vi "Connect.vi"(8 "error in (no error)":errorcluster, 11 "PicoScope 3000a in":refnum<class "PicoScope 3000a.lvclass">) -> (0 "error out":errorcluster, 3 "PicoScope 3000a out":refnum<class "PicoScope 3000a.lvclass">)   [LabVIEW 2018, in "PicoScope 3000a.lvlib" / "PicoScope 3000a.lvclass"]
doc: "This Override method is used initiative the communication session with the Oscope instrument."
uses:
  PicoScope 3000a.lvclass
  PicoScope 3000a.lvclass/PicoScope 3000a.ctl
  ps3000a.dll
  LWS SLA-070/Distro/Projects/12170 Luminar LWS Base/Source/PPLs/Oscilloscope.lvlibp/Oscilloscope.lvclass
  C:/Projects/LWS SLA-070/Distro/Projects/12170 Luminar LWS Base/Source/PPLs/Oscilloscope.lvlibp/Oscilloscope.lvclass
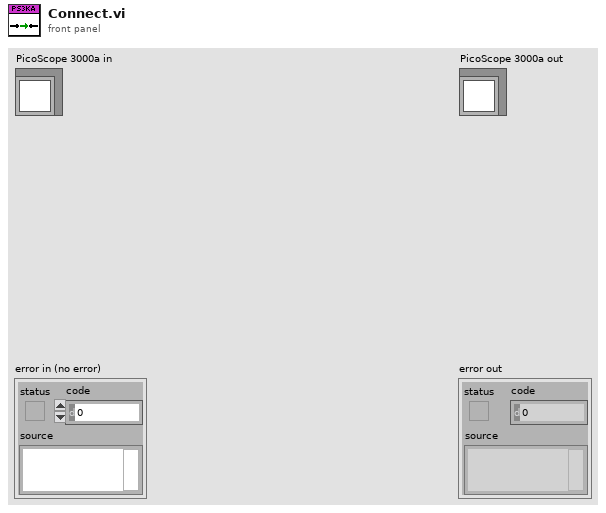
[diagram p1: front panel]
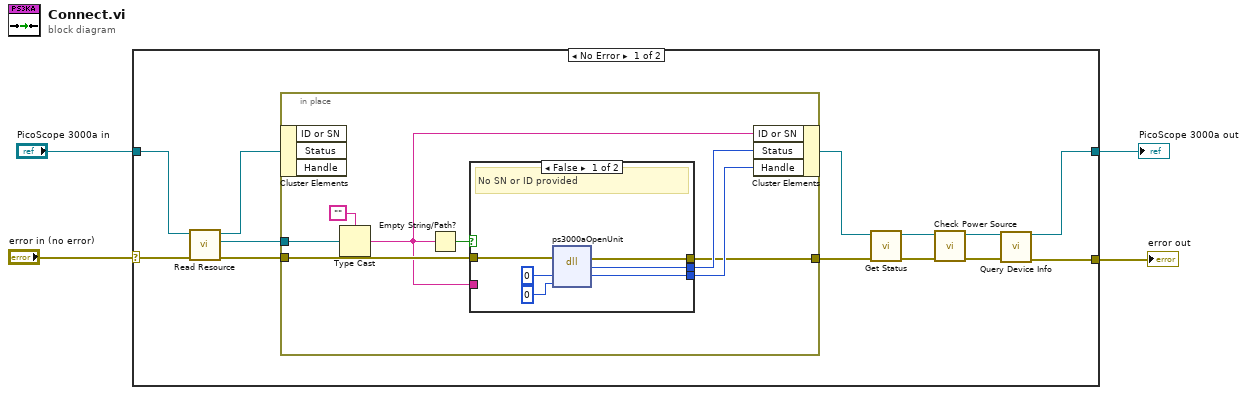
[diagram p0: block diagram]
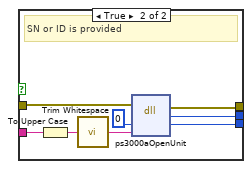
[diagram p2: hidden frame]
diagram:
  n1 = case shown="No Error" "error in (no error)" {
    selector: "error in (no error)" -> [w8 w41]
    tunnel: "PicoScope 3000a in" -> [w9 w40]
    tunnel: [w15 w40] -> w3
    tunnel: [w14 w41] -> w1
    frame No Error {
      n2 = call "Read Resource.vi"("error in (no error)"=w8, "Oscilloscope in"=w9) -> ("error out"=w7:errorcluster, "Resource"=w5:refnum<visa-resource-name>, "Oscilloscope out"=w6:refnum<class "PicoScope 3000a.lvclass">)  [unwired: 7 in]
      n3 = in-place {
        in-place-border: w7 -> [w24]
        in-place-border: [w21] -> w13
        in-place-border: w5 -> [w20]
        n4 = in-place-cluster #1(w6) -> ()  [unwired: 3 out]
        n5 = Type Cast(type="", x=w20) -> (*(type *) &x=w18:string)
        n6 = Empty String/Path?(string/path=w18) -> (empty?=w25:bool)
        n7 = case shown="False" w25 {
          tunnel: w24 -> [w31 w38]
          tunnel: [w29 w37] -> w21
          tunnel: [w28 w34] -> w22
          tunnel: [w27 w36] -> w23
          tunnel: w18 -> [_ w33]
          frame False {
            # "No SN or ID provided"
            n8 = dll-call lib="ps3000a.dll" fn="ps3000aOpenUnit" label="ps3000.dll:_ps3000_open_unit"(error in=w31, "handle"=i16 0, "serial"=i8 0) -> (error out=w29:errorcluster, "PICO_STATUS"=w28:i32, "handle"=w27:i16)  [unwired: 3 in, 1 out]
          }
          frame True {
            # "SN or ID is provided"
            n9 = To Upper Case(1:w33) -> (0:w35:string)
            n10 = call <vilib>:"Trim Whitespace.vi"("string"=w35) -> ("trimmed string"=w32:string)  [unwired: 1 in]
            n11 = dll-call lib="ps3000a.dll" fn="ps3000aOpenUnit" label="ps3000.dll:_ps3000_open_unit"(error in=w38, "handle"=i16 0, "serial"=w32) -> (error out=w37:errorcluster, "PICO_STATUS"=w34:i32, "handle"=w36:i16)  [unwired: 3 in, 1 out]
          }
        }
        n12 = in-place-cluster #1("ID or SN"=w18, "Status"=w22, "Handle"=w23) -> (w11:refnum<class "PicoScope 3000a.lvclass">)
      }
      n13 = call-dynamic "Get Status.vi"("error in (no error)"=w13, "PicoScope 3000a in"=w11) -> ("error out"=w12:errorcluster, "PicoScope 3000a out"=w10:refnum<class "PicoScope 3000a.lvclass">)  [unwired: 7 in, 1 out]
      n14 = call "Check Power Source.vi"("error in (no error)"=w12, "PicoScope 3000a in"=w10) -> ("error out"=w16:errorcluster, "PicoScope 3000a out"=w17:refnum<class "PicoScope 3000a.lvclass">)  [unwired: 8 in]
      n15 = call "Query Device Info.vi"("PicoScope 3000a in"=w17, "error in (no error)"=w16) -> ("PicoScope 3000a out"=w15:refnum<class "PicoScope 3000a.lvclass">, "error out"=w14:errorcluster)  [unwired: 12 in]
    }
    frame Error {
    }
  }
  "error out" <- w1
  "PicoScope 3000a out" <- w3
